vi "Dispose.vi"(8 "error in (no error)":errorcluster, 11 "Canvas in":refnum<class "Drawer .Net.lvclass">) -> (0 "error out":errorcluster)   [LabVIEW 2020, in "Glyph .NET.lvlib" / "Drawer .Net.lvclass"]
uses:
  Drawer .Net.lvclass
  Drawer .Net.lvclass/Drawer .Net.ctl
  System.Drawing
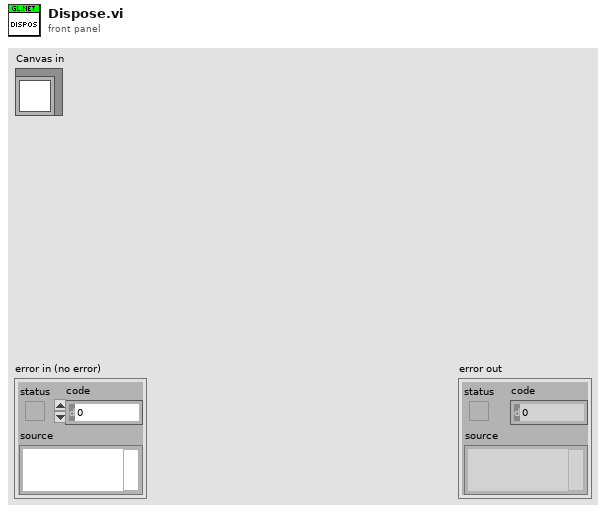
[diagram p1: front panel]
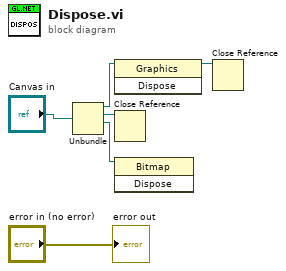
[diagram p0: block diagram]
diagram:
  n1 = Unbundle("Canvas in") -> (w5:refnum<k24>, w1:refnum<k24>, w3:refnum<k24>)  [unwired: 1 out]
  n2 = invoke class="Graphics" method="Dispose"(reference=w5) -> (reference out=w4:refnum<k24>)  [unwired: 2 in, 2 out]
  n3 = Close Reference(reference=w1) -> ()  [unwired: 1 in, 1 out]
  n4 = invoke class="Bitmap" method="Dispose"(reference=w3) -> ()  [unwired: 2 in, 3 out]
  n5 = Close Reference(reference=w4) -> ()  [unwired: 1 in, 1 out]
  "error out" <- "error in (no error)"
